vi "ExTestAdvDispPseudoColor.vi"() -> ()   [LabVIEW 2010]
panel:
  out "Array":i32[](array[numeric])
  in  "Full File Name":path
  out "error out":errorcluster
  in  "error in (no error)":errorcluster
  in  "SITKFULLDISPLAYLib.SITKFullDisplay":refnum<k7>(container)
  # "Browse match pattern is set to *.tif.  Modify this if different file type is needed."
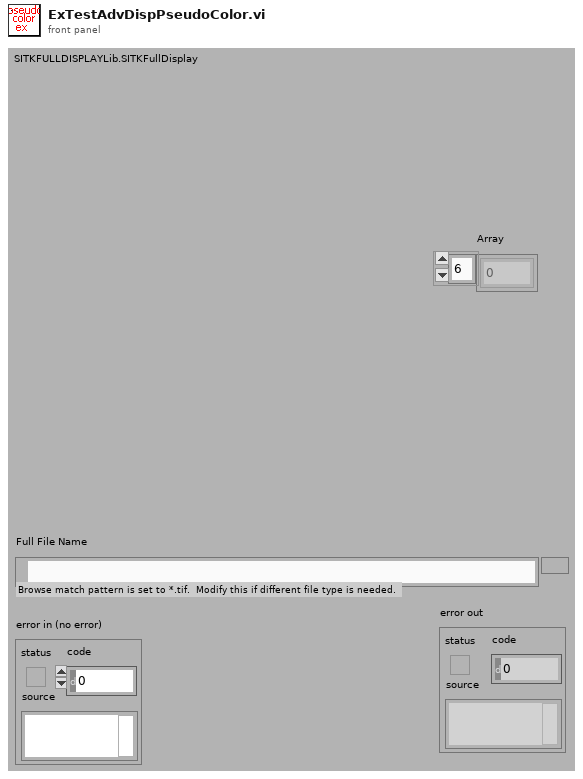
[diagram p1: front panel]
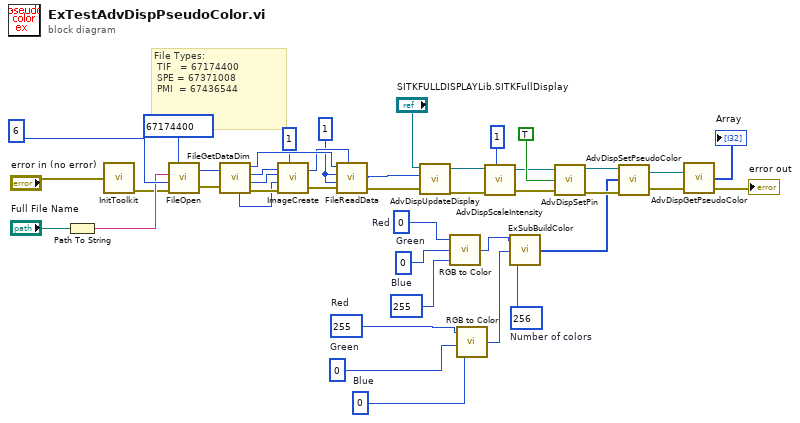
[diagram p0: block diagram]
diagram:
  w8 = 256  # Number of colors
  w12 = 0  # Blue
  w10 = 0  # Green
  w11 = 255  # Red
  w16 = 255  # Blue
  w15 = 0  # Green
  w14 = 0  # Red
  w18 = 1
  # "File Types:\n TIF   = 67174400\n SPE = 67371008\n PMI  = 67436544"
  n1 = Path To String(path="Full File Name") -> (string=w39:string)
  n2 = call <userlib>:"InitToolkit.vi"("error in"="error in (no error)") -> ("error out"=w32:errorcluster)
  n3 = call <userlib>:"FileOpen.vi"("error in"=w32, "File Operations"=6, "FileName"=w39, "File Type"=67174400) -> ("error out"=w38:errorcluster, "File Handle"=w17:u32)
  n4 = call <userlib>:"FileGetDataDim.vi"("File Handle"=w17, "error in"=w38) -> ("Data Type"=w30:u32, "File Handle"=w36:u32, "X dim"=w28:u32, "Y dim"=w29:u32, "error out"=w37:errorcluster)  [unwired: 1 out]
  n5 = call <userlib>:"ImageCreate.vi"("X dimension"=w28, "Y dimension"=w29, "Data Type"=w30, "error in"=w37, "Number Of Frames"=1) -> ("Image Handle"=w34:u32, "error out"=w35:errorcluster)
  n6 = call <userlib>:"FileReadData.vi"("File Handle"=w36, "Start Frame"=w18, "End Frame"=w18, "error in"=w35, "Image Handle"=w34) -> ("Image Handle"=w21:u32, "error out"=w27:errorcluster)  [unwired: 1 out]
  n7 = call <userlib>:"AdvDispUpdateDisplay.vi"("error in (no error)"=w27, "Image Handle"=w21, "SITKFULLDISPLAYLib.SITKFullDisplay"="SITKFULLDISPLAYLib.SITKFullDisplay") -> ("error out"=w24:errorcluster, "SITKFULLDISPLAYLib.SITKFullDisplay"=w26:refnum<k7>)  [unwired: 1 in]
  n8 = call <vilib>:"RGB to Color.vi"("B"=w16, "G"=w15, "R"=w14) -> ("Color"=w13:u32)
  n9 = call <vilib>:"RGB to Color.vi"("B"=w12, "G"=w10, "R"=w11) -> ("Color"=w9:u32)
  n10 = call <userlib>:"AdvDispScaleIntensity.vi"("SITKFULLDISPLAYLib.SITKFullDisplay"=w26, "error in (no error)"=w24, "Type of Scale"=1) -> ("SITKFULLDISPLAYLib.SITKFullDisplay"=w25:refnum<k7>, "error out"=w23:errorcluster)  [unwired: 2 in]
  n11 = call "ExSubBuildColor.vi"("Count"=w8, "End Color"=w9, "Start Color"=w13) -> ("Array"=w5:i32[])
  n12 = call <userlib>:"AdvDispSetPin.vi"("SITKFULLDISPLAYLib.SITKFullDisplay"=w25, "Pin Enable"=TRUE, "error in (no error)"=w23) -> ("SITKFULLDISPLAYLib.SITKFullDisplay"=w6:refnum<k7>, "error out"=w7:errorcluster)  [unwired: 2 out]
  n13 = call <userlib>:"AdvDispSetPseudoColor.vi"("error in (no error)"=w7, "Array"=w5, "SITKFULLDISPLAYLib.SITKFullDisplay"=w6) -> ("error out"=w4:errorcluster, "SITKFULLDISPLAYLib.SITKFullDisplay"=w3:refnum<k7>)
  n14 = call <userlib>:"AdvDispGetPseudoColor.vi"("SITKFULLDISPLAYLib.SITKFullDisplay"=w3, "error in (no error)"=w4) -> ("Array"=→"Array":i32[], "error out"=→"error out":errorcluster)  [unwired: 1 out]
